vi "Read Firmware Checksum.vi"(8 "error in (no error)":errorcluster, 9 "end address (all)":u32, 10 "start address (0)":u32, 11 "VI Probe in":refnum<class "PL MKS VI Probe.lvclass">) -> (0 "error out":errorcluster, 2 "checksum":u32, 3 "VI Probe out":refnum<class "PL MKS VI Probe.lvclass">)   [LabVIEW 2015, in "PL MKS VI Probe.lvclass"]
doc: "Reads firmware checksum."
uses:
  PL MKS VI Probe.lvclass
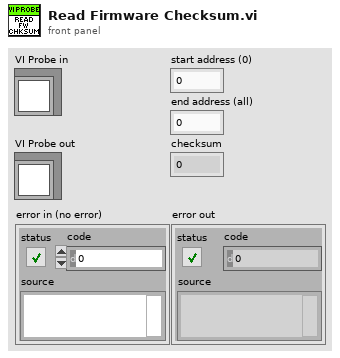
[diagram p1: front panel]
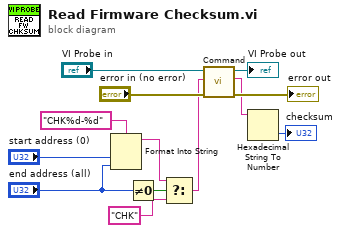
[diagram p0: block diagram]
diagram:
  n1 = Format Into String(format string="CHK%d-%d", "start address (0)", "end address (all)") -> (resulting string=w5:string)  [unwired: 2 in, 1 out]
  n2 = Not Equal To 0?(x="end address (all)") -> (x != 0?=w6:bool)
  n3 = Select(t=w5, s=w6, f="CHK") -> (s? t:f=w3:string)
  n4 = call "Command.vi"("error in (no error)"="error in (no error)", "command"=w3, "VI Probe in"="VI Probe in") -> ("error out"=→"error out":errorcluster, "response data"=w2:string, "VI Probe out"=→"VI Probe out":refnum<class "PL MKS VI Probe.lvclass">)  [unwired: 6 in]
  n5 = Hexadecimal String To Number(string=w2) -> (number=→"checksum":u32)  [unwired: 2 in, 1 out]
